vi "Main.vi"() -> ()   [LabVIEW 2012]
doc: "Demonstrates continuous waveform measurement. Spectrum is displayed in a waveform graph."
uses:
  <vilib>/Utility/file.llb/Write To Spreadsheet File (DBL).vi
  <instrlib>/Ocean Optics 2000 4000/Ocean Optics 2000 4000.lvlib
panel:
  in  "LP Filter Cuttoff Freq":dbl
  in  "Output in Polar?":bool=TRUE
  in  "ref device name":tag="Dev2"
  in  "Enable Strobe (Disabled)":bool
  in  "Spectrometer Name":refnum<visa-resource-name>
  in  "End Wavelength (< 1040 nm)":dbl format="%#_13g"
  in  "Start Wavelength (> 340 nm)":dbl format="%#_13g"
  out "standard output":string
  out "error out":errorcluster
  out "standard error":string
  in  "Reference Sample Rate (Hz)":dbl=2000.0
  in  "Time For Inner Loop (s)":dbl=2.0 caption="Time Target (s)"
  in  "Time to Run (s)":dbl format="%#_13g"
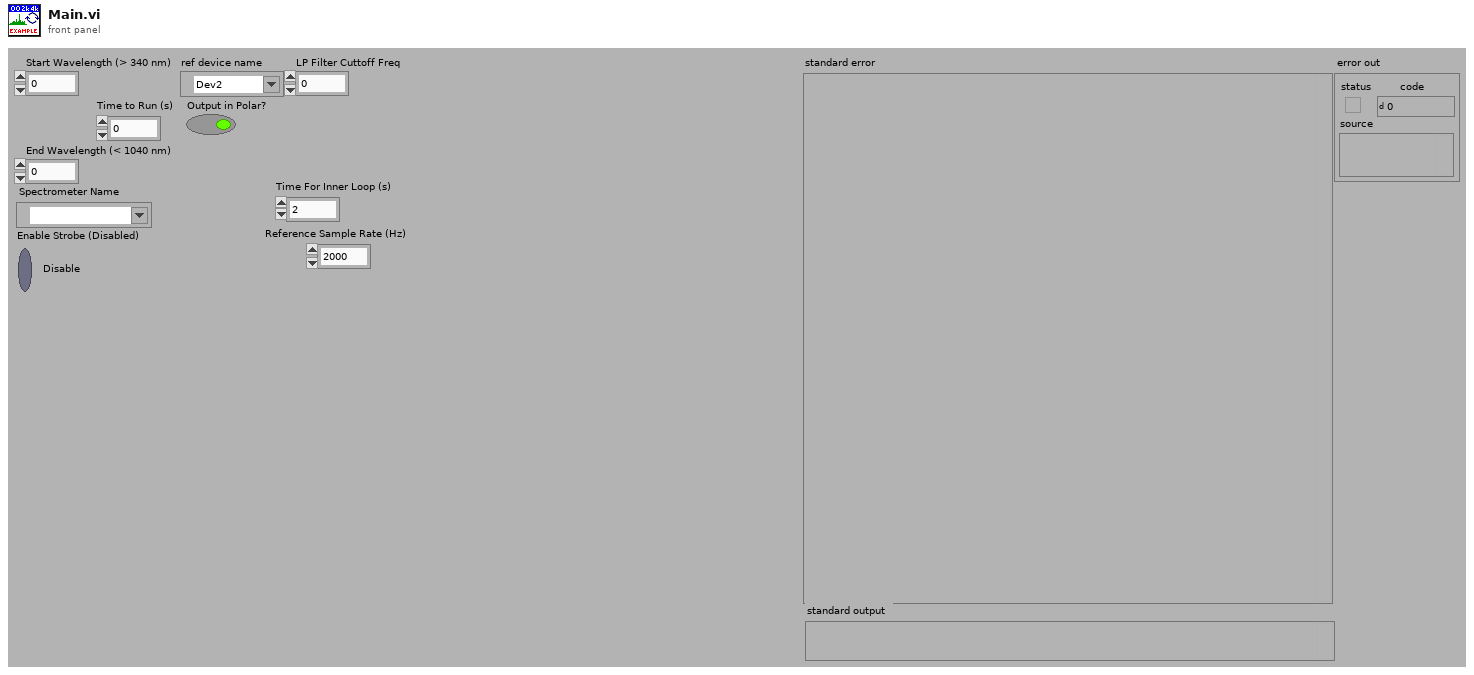
[diagram p1: front panel]
types:
  T1 = cluster{"Wavelength (nm)":dbl[], "Spectrum by Pixel Number":dbl[]}
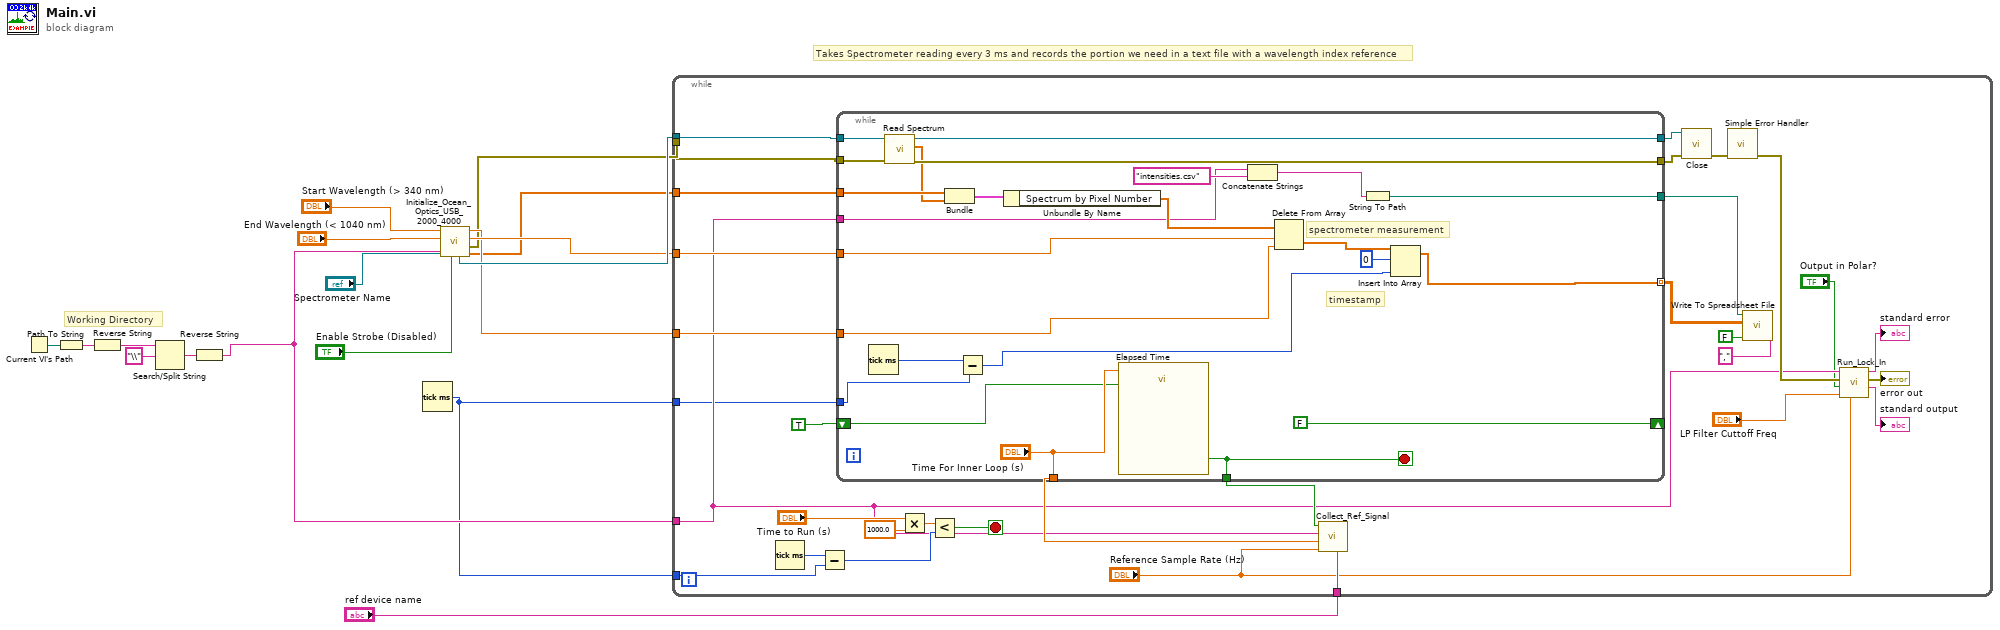
[diagram p0: block diagram]
diagram:
  # "Working Directory"
  # "Takes Spectrometer reading every 3 ms and records the portion we need in a text file with a wavelength index reference"
  n1 = Current VI's Path() -> (path=w13:path)
  n2 = Path To String(path=w13) -> (string=w17:string)
  n3 = Reverse String(1:w17) -> (0:w16:string)
  n4 = Search/Split String(string=w16, search string/char (-)="\\") -> (match + rest of string=w14:string)  [unwired: 1 in, 2 out]
  n5 = Reverse String(1:w14) -> (0:w4:string)
  n6 = Tick Count (ms)() -> (millisecond timer value=w3:u32)
  n7 = call "Initialize_Ocean_Optics_USB_2000_4000.vi"("Enable Strobe (Disabled)"="Enable Strobe (Disabled)", "VISA resource name"="Spectrometer Name", "Working Directory"=w4, "End Wavelength (< 1040 nm)"="End Wavelength (< 1040 nm)", "Start Wavelength (> 340 nm)"="Start Wavelength (> 340 nm)") -> ("Wavelength (nm)"=w5:dbl[], "error out"=w1:errorcluster, "Length of Spec Data to Keep"=w7:dbl, "Start Index of Spec Data to Keep"=w6:dbl, "VISA resource name out"=w8:refnum<visa-resource-name>)  [unwired: 2 in]
  n8 = while {
    tunnel: w8 -> [w49]
    tunnel: w1 -> [w48]
    tunnel: w5 -> [w47]
    tunnel: w6 -> [w46]
    tunnel: w7 -> [w45]
    tunnel: w4 -> [w24]
    tunnel: w3 -> [w23]
    tunnel: w3 -> [w22]
    tunnel: "ref device name" -> [w21]
    stop <- w44 stop-if-true
    n9 = Tick Count (ms)() -> (millisecond timer value=w34:u32)
    n10 = Subtract(x=w34, y=w22) -> (x-y=w32:u32)
    n11 = while {
      tunnel: [w73] -> w43
      tunnel: [w72] -> w42
      tunnel: w47 -> [w71]
      tunnel: w49 -> [w69]
      tunnel: w48 -> [w68]
      tunnel: w45 -> [w65]
      tunnel: w46 -> [w64]
      tunnel: [w57] -> w37
      tunnel: [w61] -> w33 mode=indexing
      tunnel: w23 -> [w59]
      tunnel: [w55] -> w29
      tunnel: ["Time For Inner Loop (s)"] -> w30
      shift-right: [FALSE ("Time has Elapsed")] -> _
      shift-left: TRUE ("Time has Elapsed") -> [w54]
      tunnel: w24 -> [w50]
      stop <- w55 stop-if-true
      # "spectrometer measurement"
      # "timestamp"
      n12 = Tick Count (ms)() -> (millisecond timer value=w60:u32)
      n13 = call <instrlib>:"Read Spectrum.vi"("error in (no error)"=w68, "VISA resource name"=w69) -> ("error out"=w72:errorcluster, "Spectrum by Pixel Number"=w70:dbl[], "VISA resource name out"=w73:refnum<visa-resource-name>)  [unwired: 6 in, 1 out]
      n14 = Bundle("Wavelength (nm)"=w71, "Spectrum by Pixel Number"=w70) -> (w67:T1)  [unwired: 1 out]
      n15 = Subtract(x=w60, y=w59) -> (x-y=w58:u32)
      n16 = Unbundle By Name(w67) -> ("Spectrum by Pixel Number"=w66:dbl[])
      n17 = call "Elapsed Time"("Time Target (s)"="Time For Inner Loop (s)", "Reset"=w54) -> ("Time has Elapsed"=w55:bool)  [unwired: 10 in, 7 out]
      n18 = Concatenate Strings(w50, "intensities.csv") -> (w51:string)
      n19 = Delete From Array(array=w66, length=w65, index=w64) -> (deleted portion=w63:dbl[])  [unwired: 1 out]
      n20 = String To Path(string=w51) -> (path=w57:path)
      n21 = Insert Into Array(array=w63, index=0, new element=w58) -> (w61:dbl[])
    }
    n22 = Multiply(x="Time to Run (s)", y=1000.0) -> (x*y=w40:dbl)
    n23 = Less?(x=w40, y=w32) -> (x < y?=w44:bool)
    n24 = call "Collect_Ref_Signal.vi"("ref device name"=w21, "Reference Sample Rate (Hz)"="Reference Sample Rate (Hz)", "Inner Loop Run Time"=w30, "Working Directory"=w24, "Inner Loop Ended?"=w29) -> ()  [unwired: 6 in, 1 out]
    n25 = call <instrlib>:"Close.vi"("error in (no error)"=w42, "VISA resource name"=w43) -> ("error out"=w41:errorcluster)  [unwired: 9 out]
    n26 = call <vilib>:"Simple Error Handler.vi"("error in (no error)"=w41) -> ("error out"=w28:errorcluster)  [unwired: 1 in, 7 out]
    n27 = call-poly <vilib>:"Write To Spreadsheet File.vi"("delimiter (\\t)"=",", "append to file? (new file:F)"=FALSE, "2D data"=w33, "file path (dialog if empty)"=w37) -> ()  [unwired: 4 in, 1 out]
    n28 = call "Run_Lock_In.vi"("Reference Signal Sampling Rate"="Reference Sample Rate (Hz)", "LP Filter Cuttoff Freq"="LP Filter Cuttoff Freq", "Output in Polar?"="Output in Polar?", "error in (no error)"=w28, "Working Directory"=w24) -> ("standard output"=→"standard output":string, "error out"=→"error out":errorcluster, "standard error"=→"standard error":string)  [unwired: 4 in]
  }
